vi "SIM BDF Check Convergence.vi"(0 "f(y)":dbl[](array[numeric]), 1 "y":dbl[](array[numeric]), 2 "err tolerance":dbl[](array[numeric]), 3 "step size":dbl, 4 "BDF data":T1) -> (5 "y next":dbl[](array[numeric]), 6 "converged?":bool, 7 "Newton Error?":bool)   [LabVIEW 2017]
uses:
  SIM BDF data.ctl
  SIM Factored Matrix.ctl
  SIM BDF stages.ctl
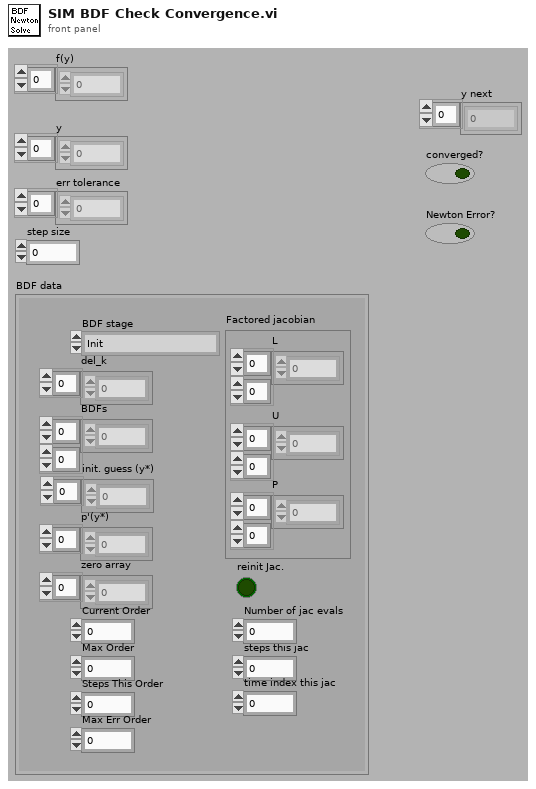
[diagram p1: front panel]
types:
  T1 = typedef "SIM BDF data.ctl" = cluster{"BDFs":dbl[][], "init. guess (y*)":dbl[], "p'(y*)":dbl[], "Factored jacobian":T2, "zero array":dbl[], "reinit Jac.":bool, "BDF stage":T3, "steps this jac":i32, "time index this jac":i32, "Number of jac evals":i32, "del_k":dbl[], "Current Order":i32, "Max Order":i32, "Steps This Order":i32, "Max Err Order":i32}
  T2 = typedef "SIM Factored Matrix.ctl" = cluster{"L":dbl[][], "U":dbl[][], "P":i32[][]}
  T3 = typedef "SIM BDF stages.ctl" = enum16{"Init", "Initial Guess", "Compute Jacobian", "Newton Iteration", "Eval Error", "Choose StepSize", "Reset BDFs"}
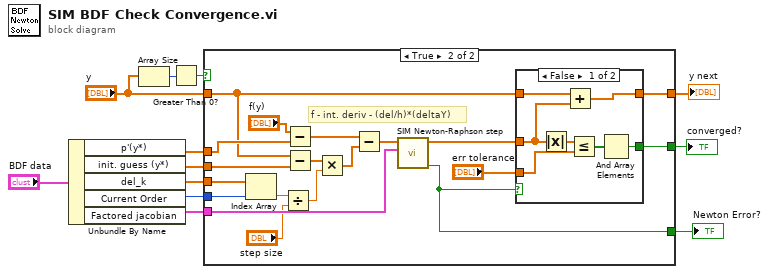
[diagram p0: block diagram]
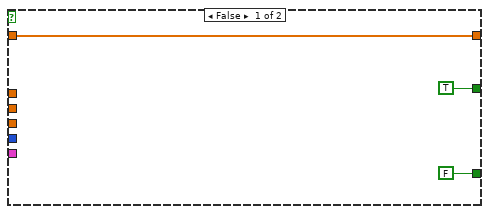
[diagram p2: hidden frame]
diagram:
  n1 = Unbundle By Name("BDF data") -> ("p'(y*)"=w9:dbl[], "init. guess (y*)"=w8:dbl[], "del_k"=w10:dbl[], "Current Order"=w7:i32, "Factored jacobian"=w11:T2)
  n2 = Array Size(array="y") -> (size(s)=w2:i32)
  n3 = Greater Than 0?(x=w2) -> (x > 0?=w3:bool)
  n4 = case shown="True" w3 {
    tunnel: w11 -> [_ w33]
    tunnel: w10 -> [_ w32]
    tunnel: w9 -> [_ w31]
    tunnel: w8 -> [_ w30]
    tunnel: w7 -> [_ w22]
    tunnel: "y" -> [w15 w21]
    tunnel: [w15 w20] -> w6
    tunnel: [TRUE w17] -> w5
    tunnel: [FALSE ("Newton Error?") w16] -> w4
    frame False {
    }
    frame True {
      # "f - int. deriv - (del/h)*(deltaY)"
      n5 = Index Array(array=w32, index=w22) -> (element=w26:dbl)
      n6 = Divide(x=w26, y="step size") -> (x/y=w28:dbl)
      n7 = Subtract(x="f(y)", y=w31) -> (x-y=w24:dbl[])
      n8 = Subtract(x=w21, y=w30) -> (x-y=w23:dbl[])
      n9 = Multiply(x=w23, y=w28) -> (x*y=w25:dbl[])
      n10 = Subtract(x=w24, y=w25) -> (x-y=w34:dbl[])
      n11 = call "SIM Newton-Raphson step.vi"("Factored Jacobian"=w33, "F(y_current)"=w34) -> ("Newton Error?"=w16:bool, "y next minus y current"=w19:dbl[])  [unwired: 8 out]
      n12 = case shown="False" w16 {
        tunnel: w21 -> [w41 w42]
        tunnel: [w40 w42] -> w20
        tunnel: w19 -> [w39 _]
        tunnel: "err tolerance" -> [w37 _]
        tunnel: [w35 _] -> w17
        frame False {
          n13 = Absolute Value(x=w39) -> (abs(x)=w38:dbl[])
          n14 = Add(x=w41, y=w39) -> (x+y=w40:dbl[])
          n15 = Less Or Equal?(x=w38, y=w37) -> (x <= y?=w36:bool[])
          n16 = And Array Elements(Boolean array=w36) -> (logical AND=w35:bool)
        }
        frame True {
        }
      }
    }
  }
  "converged?" <- w5
  "y next" <- w6
  "Newton Error?" <- w4
